vi "Setup UI.vi"(8 "error in (no error)":errorcluster, 10 "Set UI to input? (F)":bool, 11 "Pulse Gen Scan in":refnum<class "Pulse Gen Scan.lvclass">) -> (0 "error out":errorcluster, 3 "Pulse Gen Scan out":refnum<class "Pulse Gen Scan.lvclass">)   [LabVIEW 2009, in "Pulse Gen Scan.lvclass"]
doc: "Scanner::Setup is a constructor that has no parameters and faces the user. The Factory calls this VI to let the user configure this Scanner. It is dynamically dispatched in order to let the user choose the type as well as the options of the scanner."
uses:
  Pulse Gen Scan.lvclass
  Pulse Gen Scan.lvclass/Pulse Gen Scan.ctl
panel:
  out "Expected external period/frequency (text)":string="Expected external period/frequency"
  out "Desired overall period/frequency (text)":string="Desired overall period/frequency"
  in  "Trigger Mode":bool caption="External"
  in  "template: Rabi scan":bool
  out "Array of Ch2 times used":dbl[unit][](array[numeric])
  in  "Repeat sequence,\ncentered on 3T/4?":bool
  in  "Ch1 pulses centered \non trigger T/4?":enum32{"none", "first", "second"}(radio)
  out "time per bit":dbl[unit]
  out "Array of Ch1 times used":dbl[unit][](array[numeric])
  in  "period/frequency":bool
  in  "template: spin echo scan":bool
  in  "template: pump/probe scan":bool
  in  "template: pulse width scan":bool
  in  "indCh2width?":bool
  in  "indChdelay?":bool
  in  "indWidth3?":bool
  in  "indDelay3?":bool
  in  "ind3Width2?":bool
  in  "indDelay2?":bool
  in  "indWidth1?":bool
  in  "indDelay1?":bool
  in  "Overall frequency":dbl[unit]
  in  "Overall period":dbl[unit]
  in  "Ch2width":dbl[unit]
  in  "Ch2delay":dbl[unit]
  in  "width3":dbl[unit]
  in  "delay3":dbl[unit]
  in  "width2":dbl[unit]
  in  "delay2":dbl[unit]
  in  "width1":dbl[unit]
  in  "delay1":dbl[unit]
  in  "Send conds for first point to PG":bool
  out "Ch 1 Digital Waveform Graph":digitalwaveform(graph)
  out "Ch1 output string":string
  out "Ch2 output string":string
  out "Ch 2 Digital Waveform Graph":digitalwaveform(graph)
  in  "Ch2 Delay relative \nto end of Ch1?":bool
  # "ind. variable?"
  # "PURE VIRTUAL\nMETHOD CALLED!"
  # "Internal"
  # "Pulse Gen Scan"
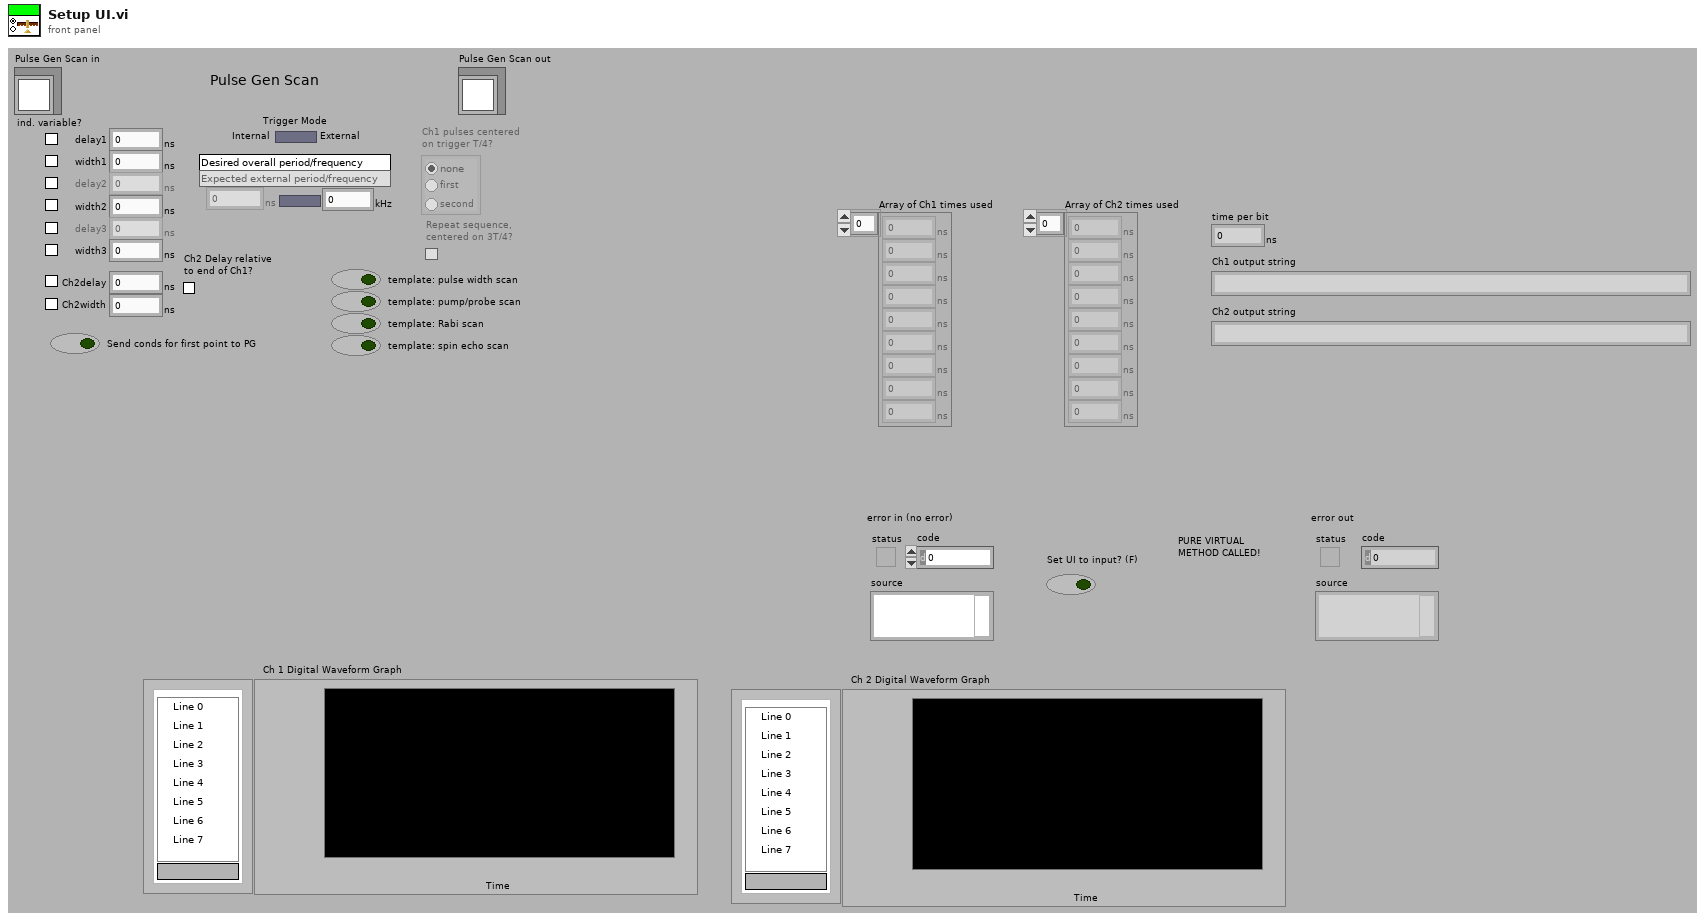
[diagram p1: front panel]
types:
  T1 = typedef "Scanner.lvclass/Range.ctl" = cluster{"xi":dbl, "xf":dbl, "dx":dbl, "Return to...?":bool, "Return to":dbl}
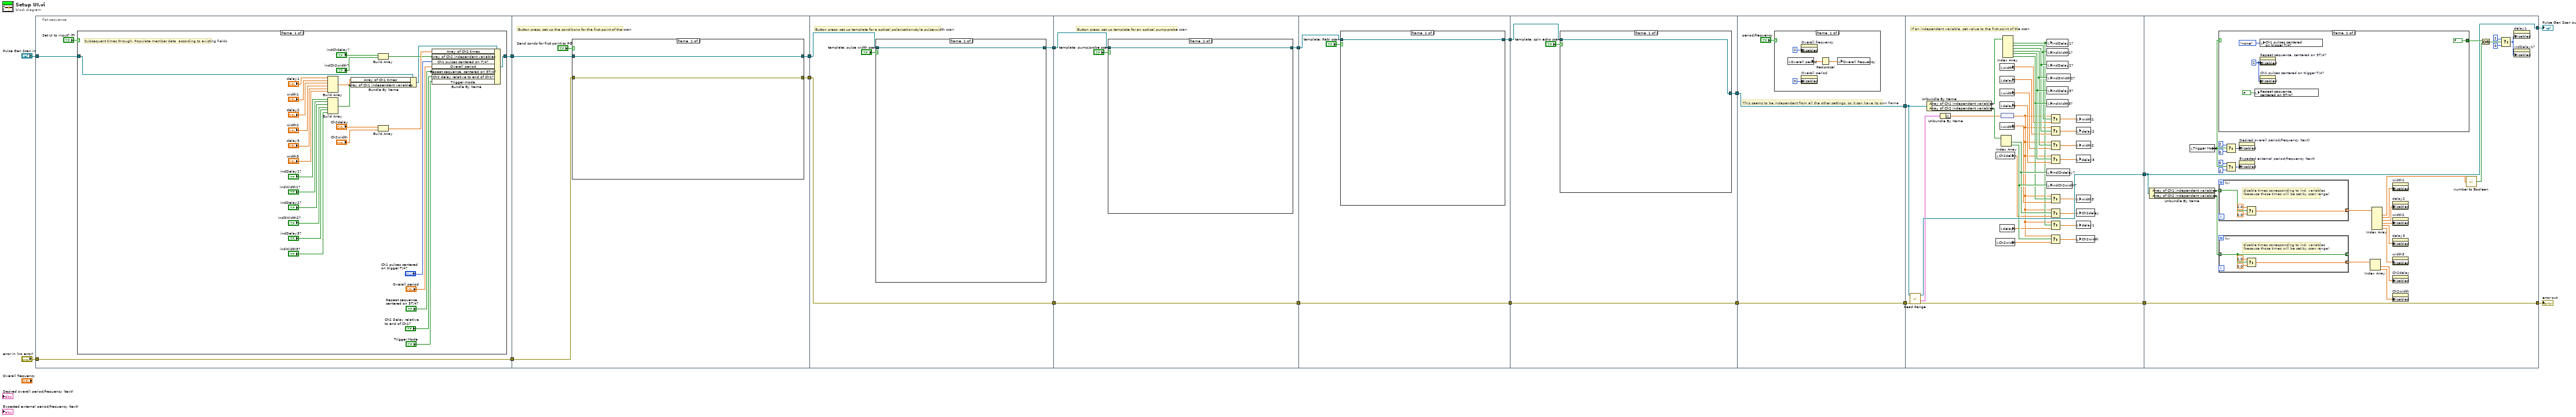
[diagram p0: block diagram]
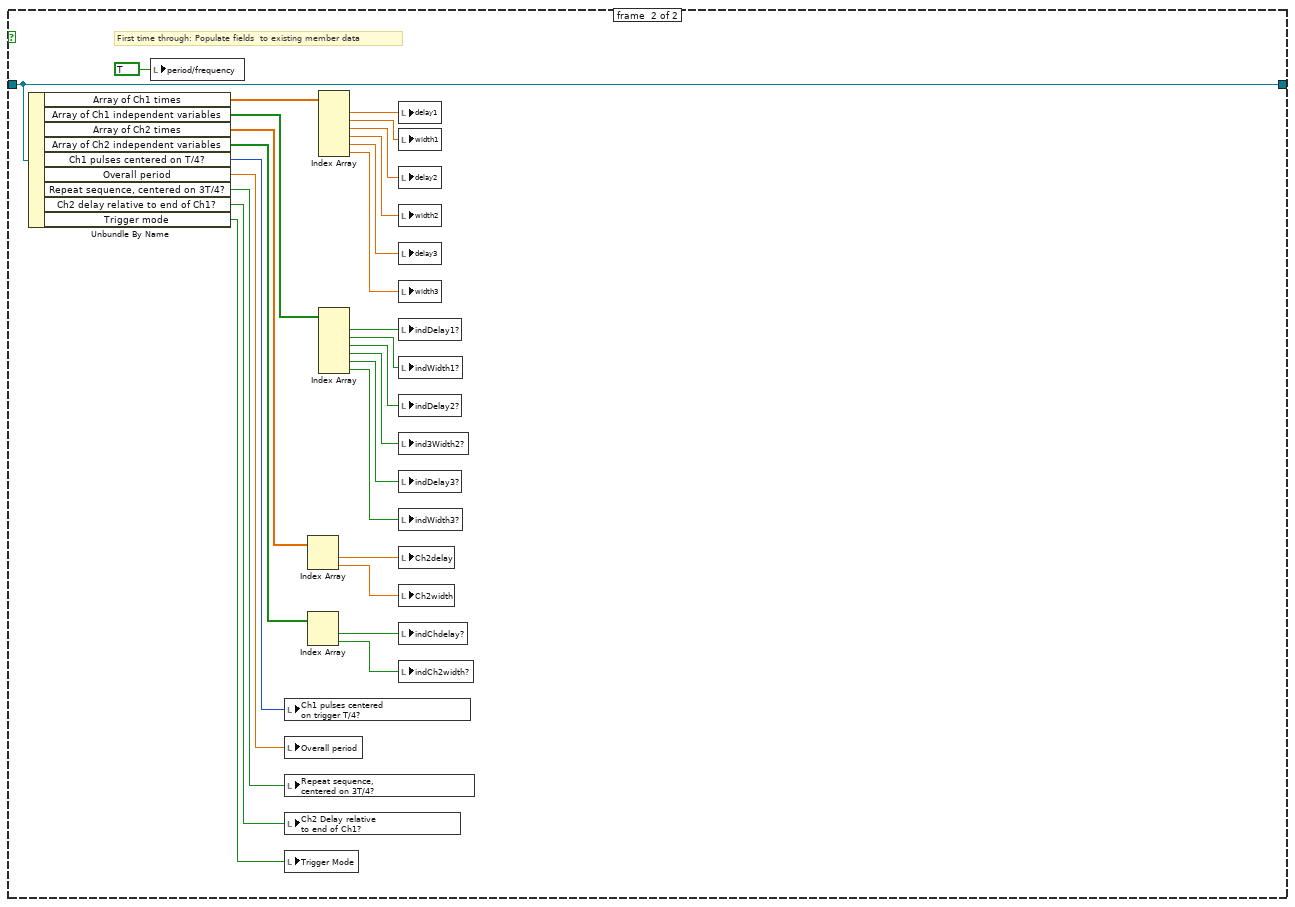
[diagram p2: hidden frame]
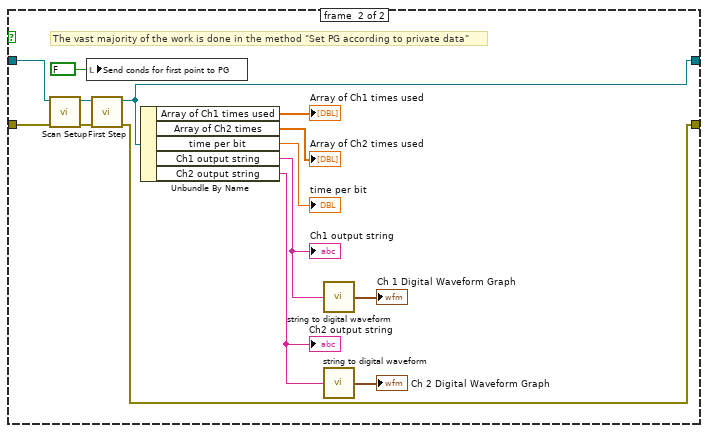
[diagram p3: hidden frame]
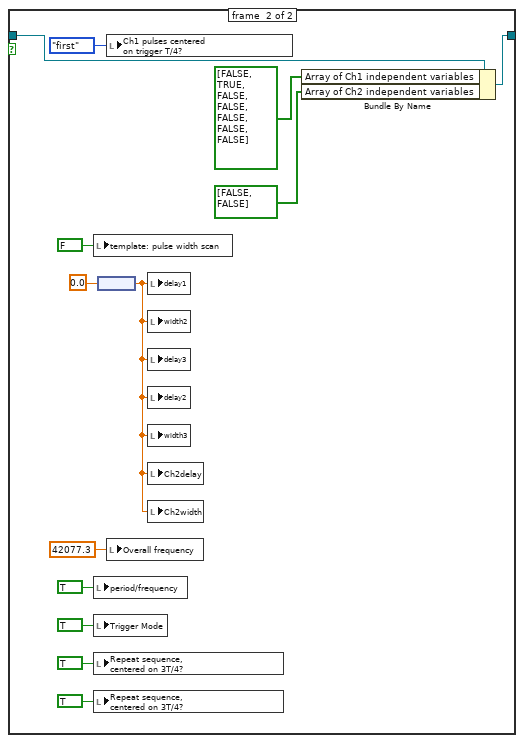
[diagram p4: hidden frame]
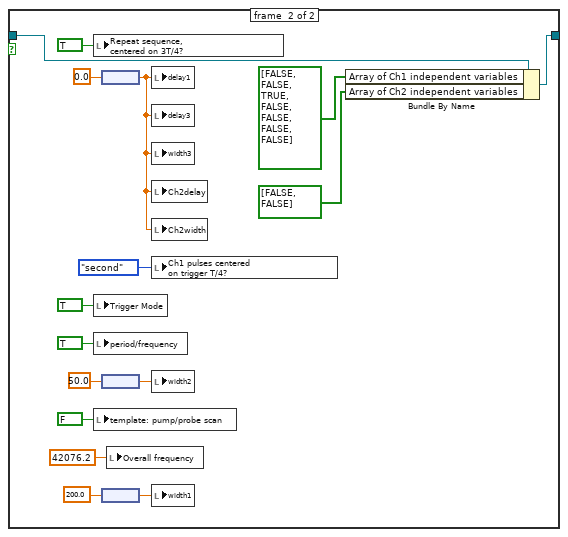
[diagram p5: hidden frame]
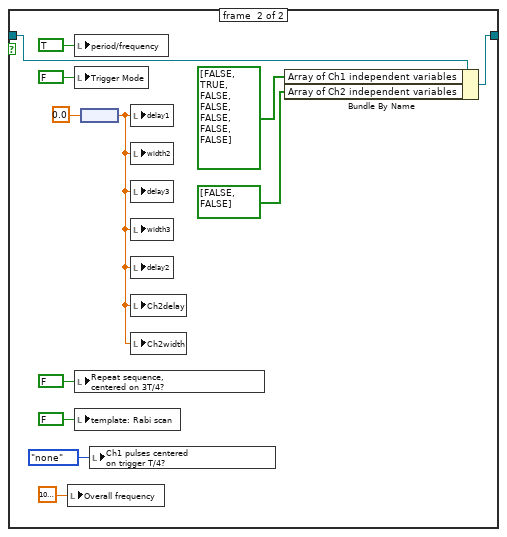
[diagram p6: hidden frame]
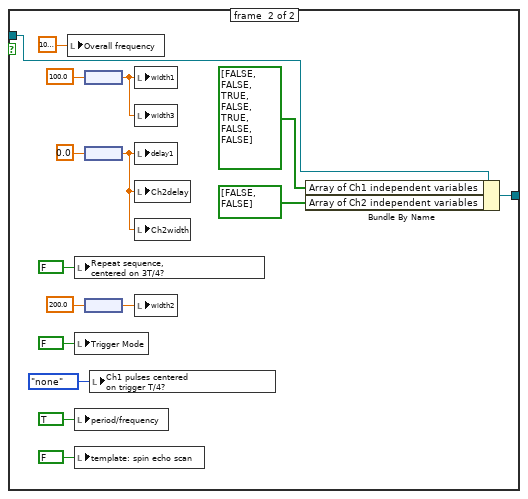
[diagram p7: hidden frame]
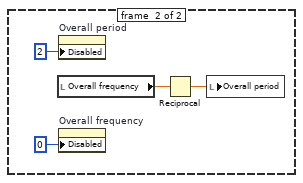
[diagram p8: hidden frame]
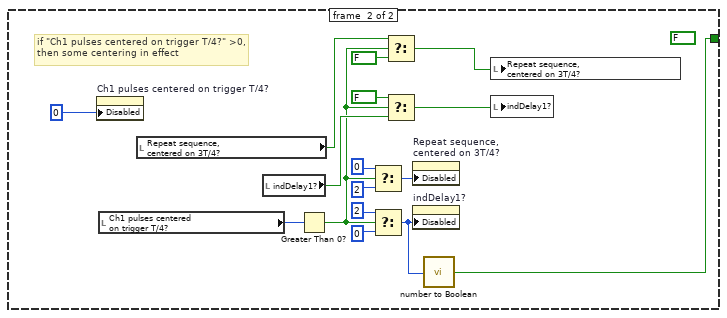
[diagram p9: hidden frame]
diagram:
  n1 = flat-sequence {
    tunnel: "error in (no error)" -> [w22]
    tunnel: "Pulse Gen Scan in" -> [w23]
    tunnel: [w21] -> w9
    tunnel: [w22] -> w8
    tunnel: w9 -> [w84]
    tunnel: [w82] -> w16
    tunnel: w8 -> [w83]
    tunnel: [w81] -> w15
    tunnel: w16 -> [w102]
    tunnel: [w103] -> w20
    tunnel: [w101] -> w19
    tunnel: w15 -> [w103]
    tunnel: [w119] -> w13
    tunnel: [w121] -> w11
    tunnel: w20 -> [w121]
    tunnel: w19 -> [w120]
    tunnel: w13 -> [w142]
    tunnel: [w141] -> w12
    tunnel: w11 -> [w143]
    tunnel: [w143] -> w10
    tunnel: w12 -> [w158]
    tunnel: [w157] -> w7
    tunnel: w10 -> [w159]
    tunnel: [w159] -> w6
    tunnel: w7 -> [w180]
    tunnel: [w180] -> w5
    tunnel: w6 -> [w179]
    tunnel: [w179] -> w3
    tunnel: w5 -> [w221]
    tunnel: [w220] -> w4
    tunnel: w3 -> [w219]
    tunnel: [w218] -> w2
    tunnel: w4 -> [w223]
    tunnel: w2 -> [w224]
    tunnel: [w224] -> w14
    tunnel: [w223] -> w1
    frame #0 {
      n2 = case shown="False" "Set UI to input? (F)" {
        tunnel: w23 -> [w30 w55]
        tunnel: [w31 w55] -> w21
        frame #0 {
          # "Subsequent times through: Populate member data  according to existing fields"
          n3 = Build Array("delay1", "width1", "delay2", "width2", "delay3", "width3") -> (w29:dbl[unit][])
          n4 = Build Array("indDelay1?", "indWidth1?", "indDelay2?", "ind3Width2?", "indDelay3?", "indWidth3?") -> (w28:bool[])
          n5 = Bundle By Name(cluster=w30, "Array of Ch1 times"=w29, "Array of Ch1 independent variables"=w28) -> (w27:refnum<class "Pulse Gen Scan.lvclass">)
          n6 = Build Array("indChdelay?", "indCh2width?") -> (w34:bool[])
          n7 = Build Array("Ch2delay", "Ch2width") -> (w37:dbl[unit][])
          n8 = Bundle By Name(cluster=w27, "Array of Ch2 times"=w37, "Array of Ch2 independent variables"=w34, "Ch1 pulses centered on T/4?"="Ch1 pulses centered \non trigger T/4?", "Overall period"="Overall period", "Repeat sequence, centered on 3T/4?"="Repeat sequence,\ncentered on 3T/4?", "Ch2 delay relative to end of Ch1?"="Ch2 Delay relative \nto end of Ch1?", "Trigger mode"="Trigger Mode") -> (w31:refnum<class "Pulse Gen Scan.lvclass">)
        }
        frame #1 {
          # "First time through: Populate fields  to existing member data"
          n9 = Unbundle By Name(w55) -> ("Array of Ch1 times"=w67:dbl[unit][], "Array of Ch1 independent variables"=w61:bool[], "Array of Ch2 times"=w66:dbl[unit][], "Array of Ch2 independent variables"=w60:bool[], "Ch1 pulses centered on T/4?"=w58:enum32{"none", "first", "second"}, "Overall period"=w59:dbl[unit], "Repeat sequence, centered on 3T/4?"=w57:bool, "Ch2 delay relative to end of Ch1?"=w56:bool, "Trigger mode"=w54:bool)
          n10 = local write "period/frequency"(TRUE) -> ()
          n11 = local write "Ch1 pulses centered \non trigger T/4?"(w58) -> ()
          n12 = local write "Overall period"(w59) -> ()
          n13 = local write "Repeat sequence,\ncentered on 3T/4?"(w57) -> ()
          n14 = local write "Ch2 Delay relative \nto end of Ch1?"(w56) -> ()
          n15 = local write "Trigger Mode"(w54) -> ()
          n16 = Index Array(array=w66) -> (element #1=w65:dbl[unit], element #2=w64:dbl[unit])  [unwired: 2 in]
          n17 = Index Array(array=w60) -> (element #1=w63:bool, element #2=w62:bool)  [unwired: 2 in]
          n18 = Index Array(array=w67) -> (element #1=w79:dbl[unit], element #2=w78:dbl[unit], element #3=w77:dbl[unit], element #4=w76:dbl[unit], element #5=w75:dbl[unit], element #6=w74:dbl[unit])  [unwired: 6 in]
          n19 = Index Array(array=w61) -> (element #1=w68:bool, element #2=w69:bool, element #3=w70:bool, element #4=w71:bool, element #5=w72:bool, element #6=w53:bool)  [unwired: 6 in]
          n20 = local write "delay1"(w79) -> ()
          n21 = local write "width1"(w78) -> ()
          n22 = local write "delay2"(w77) -> ()
          n23 = local write "width2"(w76) -> ()
          n24 = local write "delay3"(w75) -> ()
          n25 = local write "width3"(w74) -> ()
          n26 = local write "indDelay1?"(w68) -> ()
          n27 = local write "indWidth1?"(w69) -> ()
          n28 = local write "indDelay2?"(w70) -> ()
          n29 = local write "ind3Width2?"(w71) -> ()
          n30 = local write "indDelay3?"(w72) -> ()
          n31 = local write "indWidth3?"(w53) -> ()
          n32 = local write "Ch2delay"(w65) -> ()
          n33 = local write "Ch2width"(w64) -> ()
          n34 = local write "indChdelay?"(w63) -> ()
          n35 = local write "indCh2width?"(w62) -> ()
        }
      }
    }
    frame #1 {
      # "Button press: set up the conditions for the first point of the scan"
      n36 = case shown="True" "Send conds for first point to PG" {
        tunnel: [w86 w92] -> w82
        tunnel: [w85 w91] -> w81
        tunnel: w84 -> [w86 w90]
        tunnel: w83 -> [w85 w89]
        frame #0 {
        }
        frame #1 {
          # "The vast majority of the work is done in the method \"Set PG according to private data\""
          n37 = call-dynamic "Scan Setup.vi"("error in (no error)"=w89, "Pulse Gen Scan in"=w90) -> ("error out"=w87:errorcluster, "Pulse Gen Scan out"=w88:refnum<class "Pulse Gen Scan.lvclass">)  [unwired: 8 out]
          n38 = local write "Send conds for first point to PG"(FALSE ("Send conds for first point to PG")) -> ()
          n39 = call-dynamic "First Step.vi"("error in (no error)"=w87, "Pulse Gen Scan.lvclass in"=w88) -> ("error out"=w91:errorcluster, "Pulse Gen Scan.lvclass out"=w92:refnum<class "Pulse Gen Scan.lvclass">)  [unwired: 8 out]
          n40 = Unbundle By Name(w92) -> ("Array of Ch1 times used"=→"Array of Ch1 times used":dbl[unit][], "Array of Ch2 times"=→"Array of Ch2 times used":dbl[unit][], "time per bit"=→"time per bit":dbl[unit], "Ch1 output string"=w97:string, "Ch2 output string"=w96:string)
          "Ch1 output string" <- w97
          "Ch2 output string" <- w96
          n41 = call "string to digital waveform.vi"("String"=w97) -> ("digital waveform"=→"Ch 1 Digital Waveform Graph":digitalwaveform)
          n42 = call "string to digital waveform.vi"("String"=w96) -> ("digital waveform"=→"Ch 2 Digital Waveform Graph":digitalwaveform)
        }
      }
    }
    frame #2 {
      # "Button press: set up template for a optical polarization-style pulse-width scan"
      n43 = case shown="True" "template: pulse width scan" {
        tunnel: w102 -> [w105 w115]
        tunnel: [w105 w114] -> w101
        frame #0 {
        }
        frame #1 {
          n44 = local write "template: pulse width scan"(FALSE) -> ()
          n45 = local write "period/frequency"(TRUE ("period/frequency")) -> ()
          n46 = local write "Trigger Mode"(TRUE ("Trigger Mode")) -> ()
          n47 = local write "Repeat sequence,\ncentered on 3T/4?"(TRUE ("Repeat sequence,\ncentered on 3T/4?")) -> ()
          n48 = local write "Repeat sequence,\ncentered on 3T/4?"(TRUE ("Repeat sequence,\ncentered on 3T/4?")) -> ()
          n49 = node(0.0) -> (w106:dbl[unit])
          n50 = local write "Ch1 pulses centered \non trigger T/4?"(enum32{"none", "first", "second"}."first" ("Pulses centered \non T/4?")) -> ()
          n51 = local write "Overall frequency"(dbl[unit] 42077.3 ("Expected frequency")) -> ()
          n52 = local write "delay1"(w106) -> ()
          n53 = local write "width2"(w106) -> ()
          n54 = local write "delay3"(w106) -> ()
          n55 = local write "delay2"(w106) -> ()
          n56 = local write "width3"(w106) -> ()
          n57 = local write "Ch2delay"(w106) -> ()
          n58 = local write "Ch2width"(w106) -> ()
          n59 = Bundle By Name(cluster=w115, "Array of Ch1 independent variables"=bool[] [FALSE, TRUE, FALSE, FALSE, FALSE, FALSE, FALSE], "Array of Ch2 independent variables"=bool[] [FALSE, FALSE]) -> (w114:refnum<class "Pulse Gen Scan.lvclass">)
        }
      }
    }
    frame #3 {
      # "Button press: set up template for an optical pump-probe scan"
      n60 = case shown="True" "template: pump/probe scan" {
        tunnel: w120 -> [w123 w133]
        tunnel: [w123 w131] -> w119
        frame #0 {
        }
        frame #1 {
          n61 = local write "Repeat sequence,\ncentered on 3T/4?"(TRUE ("Repeat sequence,\ncentered on 3T/4?")) -> ()
          n62 = local write "Trigger Mode"(TRUE ("Trigger Mode")) -> ()
          n63 = local write "period/frequency"(TRUE ("period/frequency")) -> ()
          n64 = local write "template: pump/probe scan"(FALSE) -> ()
          n65 = node(0.0) -> (w124:dbl[unit])
          n66 = node(50.0) -> (w139:dbl[unit])
          n67 = node(200.0) -> (w137:dbl[unit])
          n68 = local write "Overall frequency"(dbl[unit] 42076.2 ("Expected frequency")) -> ()
          n69 = local write "delay1"(w124) -> ()
          n70 = local write "delay3"(w124) -> ()
          n71 = local write "width3"(w124) -> ()
          n72 = local write "Ch2delay"(w124) -> ()
          n73 = local write "Ch2width"(w124) -> ()
          n74 = local write "Ch1 pulses centered \non trigger T/4?"(enum32{"none", "first", "second"}."second" ("Pulses centered \non T/4?")) -> ()
          n75 = local write "width2"(w139) -> ()
          n76 = local write "width1"(w137) -> ()
          n77 = Bundle By Name(cluster=w133, "Array of Ch1 independent variables"=bool[] [FALSE, FALSE, TRUE, FALSE, FALSE, FALSE, FALSE], "Array of Ch2 independent variables"=bool[] [FALSE, FALSE]) -> (w131:refnum<class "Pulse Gen Scan.lvclass">)
        }
      }
    }
    frame #4 {
      n78 = case shown="True" "template: Rabi scan" {
        tunnel: w142 -> [w144 w153]
        tunnel: [w144 w152] -> w141
        frame #0 {
        }
        frame #1 {
          n79 = local write "Overall frequency"(dbl[unit] 10000.0 ("Expected frequency")) -> ()
          n80 = local write "period/frequency"(TRUE ("period/frequency")) -> ()
          n81 = local write "Trigger Mode"(FALSE ("Trigger Mode")) -> ()
          n82 = local write "Repeat sequence,\ncentered on 3T/4?"(FALSE ("Repeat sequence,\ncentered on 3T/4?")) -> ()
          n83 = local write "template: Rabi scan"(FALSE) -> ()
          n84 = node(0.0) -> (w147:dbl[unit])
          n85 = local write "Ch1 pulses centered \non trigger T/4?"(enum32{"none", "first", "second"}."none" ("Pulses centered \non T/4?")) -> ()
          n86 = local write "delay1"(w147) -> ()
          n87 = local write "width2"(w147) -> ()
          n88 = local write "delay3"(w147) -> ()
          n89 = local write "width3"(w147) -> ()
          n90 = local write "delay2"(w147) -> ()
          n91 = local write "Ch2delay"(w147) -> ()
          n92 = local write "Ch2width"(w147) -> ()
          n93 = Bundle By Name(cluster=w153, "Array of Ch1 independent variables"=bool[] [FALSE, TRUE, FALSE, FALSE, FALSE, FALSE, FALSE], "Array of Ch2 independent variables"=bool[] [FALSE, FALSE]) -> (w152:refnum<class "Pulse Gen Scan.lvclass">)
        }
      }
    }
    frame #5 {
      n94 = case shown="True" "template: spin echo scan" {
        tunnel: w158 -> [w161 w170]
        tunnel: [w161 w168] -> w157
        frame #0 {
        }
        frame #1 {
          n95 = local write "Overall frequency"(dbl[unit] 10000.0 ("Expected frequency")) -> ()
          n96 = local write "Repeat sequence,\ncentered on 3T/4?"(FALSE ("Repeat sequence,\ncentered on 3T/4?")) -> ()
          n97 = local write "Trigger Mode"(FALSE ("Trigger Mode")) -> ()
          n98 = local write "period/frequency"(TRUE ("period/frequency")) -> ()
          n99 = local write "template: spin echo scan"(FALSE) -> ()
          n100 = node(100.0) -> (w177:dbl[unit])
          n101 = node(0.0) -> (w173:dbl[unit])
          n102 = node(200.0) -> (w176:dbl[unit])
          n103 = local write "Ch1 pulses centered \non trigger T/4?"(enum32{"none", "first", "second"}."none" ("Pulses centered \non T/4?")) -> ()
          n104 = local write "width1"(w177) -> ()
          n105 = local write "width3"(w177) -> ()
          n106 = local write "delay1"(w173) -> ()
          n107 = local write "Ch2delay"(w173) -> ()
          n108 = local write "Ch2width"(w173) -> ()
          n109 = local write "width2"(w176) -> ()
          n110 = Bundle By Name(cluster=w170, "Array of Ch1 independent variables"=bool[] [FALSE, FALSE, TRUE, FALSE, TRUE, FALSE, FALSE], "Array of Ch2 independent variables"=bool[] [FALSE, FALSE]) -> (w168:refnum<class "Pulse Gen Scan.lvclass">)
        }
      }
    }
    frame #6 {
      # "This seems to be independent from all the other settings, so it can have its own frame"
      n111 = case shown="True" "period/frequency" {
        frame #0 {
          n112 = local read "Overall period"() -> (w181:dbl[unit])
          n113 = property on="Overall frequency" class="DigNum (strict)"("Disabled"=2 ("f")) -> ()  [unwired: 2 in, 2 out]
          n114 = property on="Overall period" class="DigNum (strict)"("Disabled"=0) -> ()  [unwired: 2 in, 2 out]
          n115 = Reciprocal(x=w181) -> (1/x=w182:dbl[unit])
          n116 = local write "Overall frequency"(w182) -> ()
        }
        frame #1 {
          n117 = local read "Overall frequency"() -> (w186:dbl[unit])
          n118 = property on="Overall period" class="DigNum (strict)"("Disabled"=2) -> ()  [unwired: 2 in, 2 out]
          n119 = property on="Overall frequency" class="DigNum (strict)"("Disabled"=0 ("f")) -> ()  [unwired: 2 in, 2 out]
          n120 = Reciprocal(x=w186) -> (1/x=w185:dbl[unit])
          n121 = local write "Overall period"(w185) -> ()
        }
      }
    }
    frame #7 {
      # "If an independent variable, set value to the first point of the scan"
      n122 = call-dynamic "Read Range.vi"("error in (no error)"=w219, "Scanner.lvclass in"=w221) -> ("error out"=w218:errorcluster, "Range"=w217:T1, "Scanner.lvclass out"=w220:refnum<class "Pulse Gen Scan.lvclass">)  [unwired: 7 out]
      n123 = Unbundle By Name(w221) -> ("Array of Ch1 independent variables"=w192:bool[], "Array of Ch2 independent variables"=w191:bool[])
      n124 = Unbundle By Name(w217) -> ("xi"=w189:dbl)
      n125 = local read "Ch2delay"() -> (w207:dbl[unit])
      n126 = local read "Ch2width"() -> (w208:dbl[unit])
      n127 = local read "width1"() -> (w196:dbl[unit])
      n128 = local read "delay2"() -> (w199:dbl[unit])
      n129 = local read "width2"() -> (w200:dbl[unit])
      n130 = local read "delay3"() -> (w203:dbl[unit])
      n131 = local read "width3"() -> (w204:dbl[unit])
      n132 = local read "delay1"() -> (w195:dbl[unit])
      n133 = node(w189) -> (w190:dbl[unit])
      n134 = Index Array(array=w191) -> (element #1=w215:bool, element #2=w216:bool)  [unwired: 2 in]
      n135 = Index Array(array=w192) -> (element #1=w193:bool, element #2=w210:bool, element #3=w211:bool, element #4=w212:bool, element #5=w213:bool, element #6=w214:bool)  [unwired: 6 in]
      n136 = local write "indDelay1?"(w193) -> ()
      n137 = local write "indWidth1?"(w210) -> ()
      n138 = local write "indDelay2?"(w211) -> ()
      n139 = local write "ind3Width2?"(w212) -> ()
      n140 = local write "indDelay3?"(w213) -> ()
      n141 = local write "indWidth3?"(w214) -> ()
      n142 = local write "indChdelay?"(w215) -> ()
      n143 = local write "indCh2width?"(w216) -> ()
      n144 = Select(t=w190, s=w210, f=w196) -> (s? t:f=w197:dbl[unit])
      n145 = Select(t=w190, s=w211, f=w199) -> (s? t:f=w198:dbl[unit])
      n146 = Select(t=w190, s=w212, f=w200) -> (s? t:f=w201:dbl[unit])
      n147 = Select(t=w190, s=w213, f=w203) -> (s? t:f=w202:dbl[unit])
      n148 = Select(t=w190, s=w214, f=w204) -> (s? t:f=w205:dbl[unit])
      n149 = Select(t=w190, s=w215, f=w207) -> (s? t:f=w206:dbl[unit])
      n150 = Select(t=w190, s=w193, f=w195) -> (s? t:f=w194:dbl[unit])
      n151 = Select(t=w190, s=w216, f=w208) -> (s? t:f=w209:dbl[unit])
      n152 = local write "width1"(w197) -> ()
      n153 = local write "delay2"(w198) -> ()
      n154 = local write "width2"(w201) -> ()
      n155 = local write "delay3"(w202) -> ()
      n156 = local write "width3"(w205) -> ()
      n157 = local write "Ch2delay"(w206) -> ()
      n158 = local write "delay1"(w194) -> ()
      n159 = local write "Ch2width"(w209) -> ()
    }
    frame #8 {
      n160 = Unbundle By Name(w223) -> ("Array of Ch1 independent variables"=w222:bool[], "Array of Ch2 independent variables"=w241:bool[])
      n161 = local read "Trigger Mode"() -> (w226:bool)
      n162 = case shown="False" w226 {
        tunnel: [FALSE w258] -> w227
        frame #0 {
          w251 = i8 2
          n163 = local write "Repeat sequence,\ncentered on 3T/4?"(FALSE ("Repeat sequence,\ncentered on 3T/4?")) -> ()
          n164 = local write "Ch1 pulses centered \non trigger T/4?"(enum32{"none", "first", "second"}."none" ("Ch1 pulses centered \non trigger T/4?")) -> ()
          n165 = property on="Repeat sequence, centered on 3T/4?" class="Bool (strict)"("Disabled"=w251) -> ()  [unwired: 2 in, 2 out]
          n166 = property on="Ch1 pulses centered on trigger T/4?" class="RadioBtnsControl (strict)"("Disabled"=w251) -> ()  [unwired: 2 in, 2 out]
        }
        frame #1 {
          (unwired) FALSE
          # "if \"Ch1 pulses centered on trigger T/4?\" >0, \nthen some centering in effect"
          n167 = property on="Ch1 pulses centered on trigger T/4?" class="RadioBtnsControl (strict)"("Disabled"=u8 0) -> ()  [unwired: 2 in, 2 out]
          n168 = local read "Ch1 pulses centered \non trigger T/4?"() -> (w264:enum32{"none", "first", "second"})
          n169 = local read "Repeat sequence,\ncentered on 3T/4?"() -> (w262:bool)
          n170 = local read "indDelay1?"() -> (w259:bool)
          n171 = Greater Than 0?(x=w264) -> (x > 0?=w256:bool)
          n172 = Select(t=0, s=w256, f=2) -> (s? t:f=w265:i32)
          n173 = Select(t=2, s=w256, f=0) -> (s? t:f=w257:i32)
          n174 = Select(t=w262, s=w256, f=FALSE) -> (s? t:f=w263:bool)
          n175 = Select(t=FALSE, s=w256, f=w259) -> (s? t:f=w261:bool)
          n176 = property on="Repeat sequence,\ncentered on 3T/4?" class="Bool (strict)"("Disabled"=w265) -> ()  [unwired: 2 in, 2 out]
          n177 = property on="indDelay1?" class="Bool (strict)"("Disabled"=w257) -> ()  [unwired: 2 in, 2 out]
          n178 = call "number to Boolean.vi"("Numeric"=w257) -> ("Boolean"=w258:bool)
          n179 = local write "Repeat sequence,\ncentered on 3T/4?"(w263) -> ()
          n180 = local write "indDelay1?"(w261) -> ()
        }
      }
      n181 = for {
        tunnel: [w274] -> w247 mode=indexing
        tunnel: w222 -> [w273] mode=indexing
        # "disable times corresponding to ind. variables \n(because those times will be set by scan range)"
        n182 = Select(t=2.0, s=w273, f=0.0) -> (s? t:f=w274:dbl)
      }
      n183 = for {
        tunnel: [w269] -> _ mode=indexing
        tunnel: [w270] -> w242 mode=indexing
        tunnel: w241 -> [w269] mode=indexing
        # "disable times corresponding to ind. variables \n(because those times will be set by scan range)"
        n184 = Select(t=2.0, s=w269, f=0.0) -> (s? t:f=w270:dbl)
      }
      n185 = Select(t=2, s=w226, f=0) -> (s? t:f=w228:i32)
      n186 = Select(t=0, s=w226, f=2) -> (s? t:f=w229:i32)
      n187 = property on="Desired overall period/frequency (text)" class="Str"("Disabled"=w228) -> ()  [unwired: 2 in, 2 out]
      n188 = property on="Expected external period/frequency (text)" class="Str"("Disabled"=w229) -> ()  [unwired: 2 in, 2 out]
      n189 = Index Array(array=w242) -> (element #1=w240:dbl, element #2=w239:dbl)  [unwired: 2 in]
      n190 = Index Array(array=w247) -> (element #1=w238:dbl, element #2=w243:dbl, element #3=w244:dbl, element #4=w245:dbl, element #5=w246:dbl, element #6=w248:dbl)  [unwired: 6 in]
      n191 = property on="width1" class="DigNum (strict)"("Disabled"=w243) -> ()  [unwired: 2 in, 2 out]
      n192 = property on="delay2" class="DigNum (strict)"("Disabled"=w244) -> ()  [unwired: 2 in, 2 out]
      n193 = property on="width2" class="DigNum (strict)"("Disabled"=w245) -> ()  [unwired: 2 in, 2 out]
      n194 = property on="delay3" class="DigNum (strict)"("Disabled"=w246) -> ()  [unwired: 2 in, 2 out]
      n195 = property on="width3" class="DigNum (strict)"("Disabled"=w248) -> ()  [unwired: 2 in, 2 out]
      n196 = property on="Ch2delay" class="DigNum (strict)"("Disabled"=w240) -> ()  [unwired: 2 in, 2 out]
      n197 = property on="Ch2width" class="DigNum (strict)"("Disabled"=w239) -> ()  [unwired: 2 in, 2 out]
      n198 = call "number to Boolean.vi"("Numeric"=w238) -> ("Boolean"=w237:bool)
      n199 = Or(x=w227, y=w237) -> (x .or. y?=w236:bool)
      n200 = Select(t=i8 2, s=w236, f=i8 0) -> (s? t:f=w225:i8)
      n201 = property on="delay1" class="DigNum (strict)"("Disabled"=w225) -> ()  [unwired: 2 in, 2 out]
      n202 = property on="indDelay1?" class="Bool (strict)"("Disabled"=w225) -> ()  [unwired: 2 in, 2 out]
    }
  }
  "error out" <- w14
  "Pulse Gen Scan out" <- w1
